vi "Connect To Board.vi"   [LabVIEW 2021]
uses:
  wrapper/LabView/SciSDK_Labview.lvlib
types:
  T1 = cluster{"Name":string, "Board Model":string, "Handle":u64}
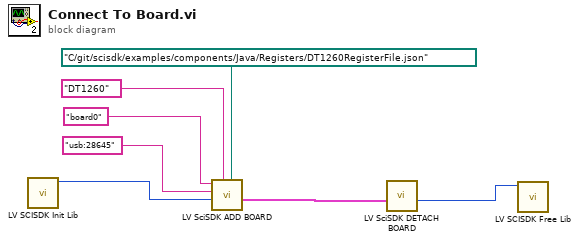
[diagram p0: block diagram]
diagram:
  n1 = call "LV SCISDK Init Lib.vi"() -> ("function return"=w7:u64)  [unwired: 11 in]
  n2 = call "LV SciSDK ADD BOARD.vi"("JsonFile"=path "C:/git/scisdk/examples/components/Java/Registers/DT1260RegisterFile.json", "Board Model"="DT1260", "SciSDK Handle"=w7, "DevicePath"="usb:28645", "Name"="board0") -> ("Board Handle Out"=w1:T1)  [unwired: 4 in, 2 out]
  n3 = call "LV SciSDK DETACH BOARD.vi"("Board Handle In"=w1) -> ("SciSDK Handle"=w2:u64)  [unwired: 9 in, 1 out]
  n4 = call "LV SCISDK Free Lib.vi"("handle"=w2) -> ()  [unwired: 9 in, 2 out]
